vi "Check_device_is_busy_set_command.vi"(10 "Json comand in":string, 11 "DEVICE":string) -> (3 "String out":string)   [LabVIEW 2015]
uses:
  Share Data/Share Variable.lvlib
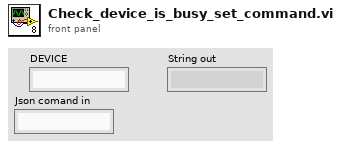
[diagram p1: front panel]
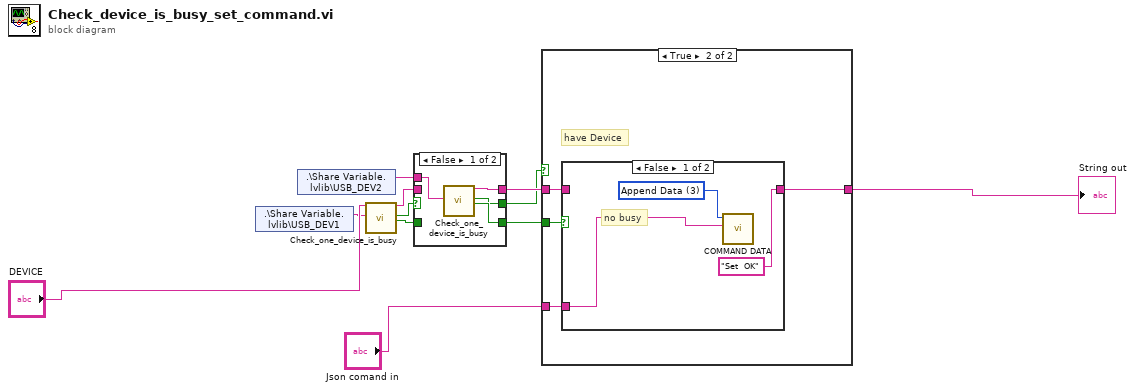
[diagram p0: block diagram]
diagram:
  n1 = shared-variable ".\\Share Variable.lvlib\\USB_DEV1"() -> (w2:string)  [unwired: 1 in, 1 out]
  n2 = shared-variable ".\\Share Variable.lvlib\\USB_DEV2"() -> (w4:string)  [unwired: 1 in, 1 out]
  n3 = call "Check_one_device_is_busy.vi"("DEVICE_SN"="DEVICE", "USB_DEV"=w2) -> ("String out"=w9:string, "Device?"=w3:bool, "BUSY"=w5:bool)  [unwired: 12 in, 3 out]
  n4 = case shown="False" w3 {
    selector: w3 -> [_ w17]
    tunnel: w4 -> [w15 _]
    tunnel: [w14 w18] -> w7
    tunnel: w5 -> [_ w18]
    tunnel: [w13 w17] -> w6
    tunnel: [w12 w16] -> w8
    tunnel: w9 -> [_ w16]
    frame False {
      n5 = call "Check_one_device_is_busy.vi"("USB_DEV"=w15) -> ("String out"=w12:string, "Device?"=w13:bool, "BUSY"=w14:bool)  [unwired: 13 in, 3 out]
    }
    frame True {
    }
  }
  n6 = case shown="True" w6 {
    tunnel: w7 -> [_ w23]
    tunnel: w8 -> [w19 w22]
    tunnel: [w19 w21] -> w10
    tunnel: "Json comand in" -> [_ w20]
    frame False {
      # "No device"
    }
    frame True {
      # "have Device"
      n7 = case shown="False" w23 {
        tunnel: w22 -> [_ w27]
        tunnel: ["Set  OK" ("String out") w27] -> w21
        tunnel: w20 -> [w24 _]
        frame False {
          w25 = u16 3 items=["Initialize Data Store", "Destroy Data Store", "Clear Data", "Append Data", "Get Last Data", "Get All Data", "Waiting - Get  Data"] ("action")
          # "no busy"
          n8 = call "COMMAND DATA.vi"("String"=w24, "action"=w25) -> ()  [unwired: 7 in, 3 out]
        }
        frame True {
          # "busy"
        }
      }
    }
  }
  "String out" <- w10
